vi "Write groupName.vi"(8 "error in (no error)":errorcluster, 10 "groupName":string, 11 "group configuration in":refnum<class "group configuration.lvclass">) -> (0 "error out":errorcluster, 3 "group configuration out":refnum<class "group configuration.lvclass">)   [LabVIEW 2013, in "group configuration.lvclass"]
uses:
  group configuration.lvclass
  Configuration Framework/serializable configuration/NISE_CEF_serializable configuration.lvclass
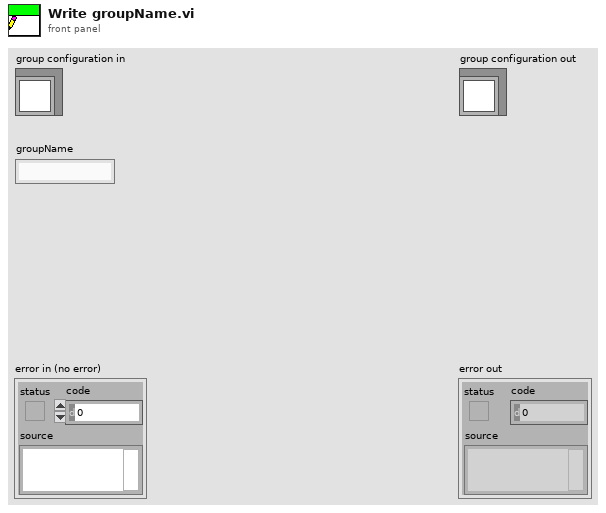
[diagram p1: front panel]
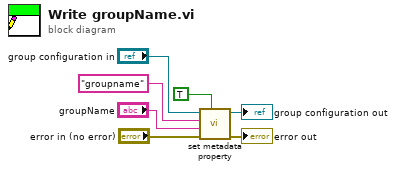
[diagram p0: block diagram]
diagram:
  n1 = call "set metadata property.vi"("overwrite?"=TRUE, "error in"="error in (no error)", "value"="groupName", "key"="groupname", "configuration in"="group configuration in") -> ("error out"=→"error out":errorcluster, "configuration out"=→"group configuration out":refnum<class "group configuration.lvclass">)  [unwired: 5 in]
